vi "Msg - Send.vi"(0 "Message":T1, 7 "High Priority?":bool, 11 "error in (no error)":errorcluster) -> (15 "error out":errorcluster)   [LabVIEW 2020, in "Template.lvlib"]
doc: "Send Messages to this Module."
uses:
  Template.lvlib
  Controls/Message.ctl
  Controls/Module - States.ctl
  Controls/Message - Queue Manager Mode.ctl
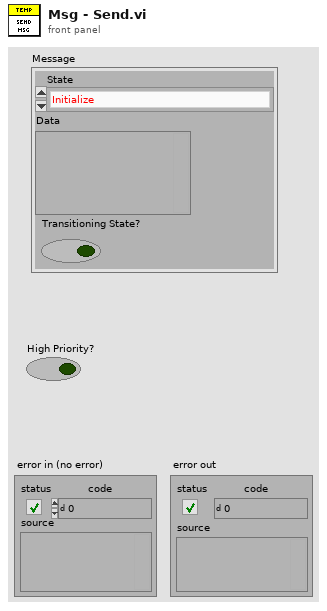
[diagram p1: front panel]
types:
  T1 = typedef "Template.lvlib/Message.ctl" = cluster{"State":T2, "Data":variant, "Transitioning State?":bool}
  T2 = typedef "Template.lvlib/Module - States.ctl" = enum16{"Initialize", "Event ", "Send data", "FP Element: Update", "FP Element: Disable/Enable", "Timer: Setup", "Terminate", "---------------Template---------------"}
  T3 = typedef "Template.lvlib/Message - Queue Manager Mode.ctl" = enum16{"Create", "Get", "Destroy"}
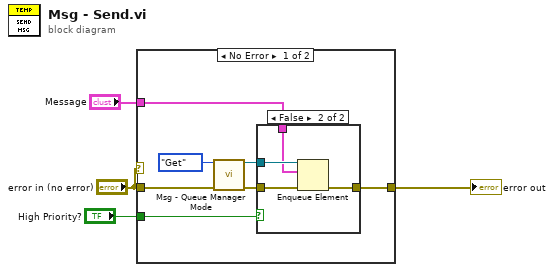
[diagram p0: block diagram]
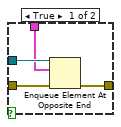
[diagram p2: hidden frame]
diagram:
  n1 = case shown="No Error" "error in (no error)" {
    tunnel: [w8 w20] -> w1
    tunnel: "error in (no error)" -> [w9 w20]
    tunnel: "Message" -> [w6 _]
    tunnel: "High Priority?" -> [w5 _]
    frame No Error {
      n2 = call "Msg - Queue Manager Mode.vi"("Mode"=Message_-_Queue_Manager_Mode."Get", "error in (no error)"=w9) -> (">>ThisModule"=w7:refnum<queue>, "error out"=w10:errorcluster)  [unwired: 11 in, 1 out]
      n3 = case shown="False" w5 {
        tunnel: w10 -> [w15 w19]
        tunnel: [w14 w18] -> w8
        tunnel: w7 -> [w13 w17]
        tunnel: w6 -> [w12 w16]
        frame True {
          n4 = Enqueue Element At Opposite End(queue=w13, element=w12, error in (no error)=w15) -> (error out=w14:errorcluster)  [unwired: 1 in, 2 out]
        }
        frame False {
          n5 = Enqueue Element(queue=w17, element=w16, error in (no error)=w19) -> (error out=w18:errorcluster)  [unwired: 1 in, 2 out]
        }
      }
    }
    frame Error {
    }
  }
  "error out" <- w1
